vi "ServoTurn.vi"(4 "error in":errorcluster, 5 "Turn to":i16(ring)=-90 items=["-90°"=-90, "0°"=0, "+90°"=90], 6 "Servo Enum":T9, 7 "PWM channel\n cluster":T8) -> (0 "error out":errorcluster, 3 "PWM Ref Out":T1)   [LabVIEW 2017]
uses:
  <vilib>/myRIO/Instrument Drivers/Onboard IO/PWM/typedefs/PWM Reference.ctl
  <vilib>/myRIO/Common/Instrument Driver Framework/Utilities/typedefs/myRIO Generic Hardware Reference.ctl
  <vilib>/myRIO/Common/Instrument Driver Framework/Utilities/typedefs/Hardware Version Enum.ctl
  <vilib>/myRIO/Common/Instrument Driver Framework/Utilities/typedefs/myRIO v1.0 Reference.ctl
  <vilib>/myRIO/Common/Instrument Driver Framework/Utilities/typedefs/Generic FPGA Reference.ctl
  <vilib>/myRIO/Common/Instrument Driver Framework/myRIO v1.0/PWM/typedefs/PWM Channels Enum.ctl
  <vilib>/myRIO/Instrument Drivers/Onboard IO/PWM/typedefs/PWM Configuration.ctl
  ServoEnumControl.ctl
  <vilib>/Utility/error.llb/Error Cluster From Error Code.vi
  <vilib>/myRIO/Common/Instrument Driver Framework/myRIO v1.0/PWM/vis/myRIO v1.0 Write PWM.vi
  <vilib>/myRIO/Instrument Drivers/Onboard IO/PWM/PWM.lvlib
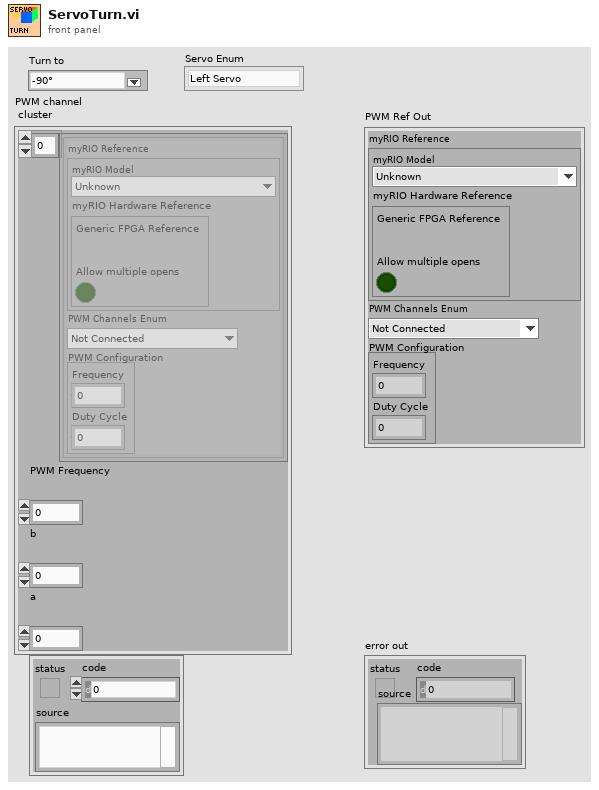
[diagram p1: front panel]
types:
  T1 = typedef "PWM.lvlib/PWM Reference.ctl" = cluster{"myRIO Reference":T2, "PWM Channels Enum":T6, "PWM Configuration":T7}
  T2 = typedef "myRIO Generic Hardware Reference.ctl" = cluster{"myRIO Model":T3, "myRIO Hardware Reference":T4}
  T3 = typedef "Hardware Version Enum.ctl" = enum16{"Unknown", "myRIO-1900", "myRIO-1950", "roboRIO", "NI ELVIS RIO CM"}
  T4 = typedef "myRIO v1.0 Reference.ctl" = cluster{"Generic FPGA Reference":T5, "Allow multiple opens":bool}
  T5 = typedef "Generic FPGA Reference.ctl" = refnum<k20>
  T6 = typedef "PWM Channels Enum.ctl" = enum16{"Not Connected", "C/PWM0", "C/PWM1", "A/PWM0", "A/PWM1", "A/PWM2", "B/PWM0", "B/PWM1", "B/PWM2", "PWM/PWM0", "PWM/PWM1", "PWM/PWM2", "PWM/PWM3", "PWM/PWM4", "PWM/PWM5", "PWM/PWM6", "PWM/PWM7", "PWM/PWM8", "PWM/PWM9"}
  T7 = typedef "PWM.lvlib/PWM Configuration.ctl" = cluster{"Frequency":dbl, "Duty Cycle":dbl}
  T8 = cluster{T1[], "PWM Frequency":dbl, "b":dbl, "a":dbl}
  T9 = typedef "ServoEnumControl.ctl" = enum16{"Left Servo", "Front Servo", "Right Servo"}
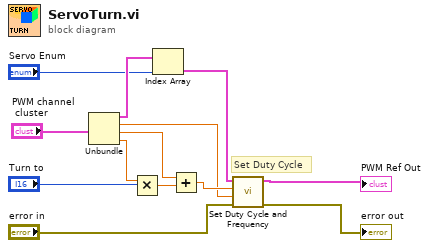
[diagram p0: block diagram]
diagram:
  # "Set Duty Cycle"
  n1 = Unbundle("PWM channel\n cluster") -> (w3:T1[], "PWM Frequency"=w4:dbl, "b"=w5:dbl, "a"=w6:dbl)
  n2 = Multiply(x=w6, y="Turn to") -> (x*y=w10:dbl)
  n3 = Index Array(array=w3, index="Servo Enum") -> (element=w1:T1)
  n4 = Add(x=w5, y=w10) -> (x+y=w9:dbl)
  n5 = call <vilib>:"Set Duty Cycle and Frequency.vi"("error in (no error)"="error in", "Frequency [Hz]"=w4, "Duty Cycle"=w9, "PWM Ref In"=w1) -> ("error out"=→"error out":errorcluster, "PWM Ref Out"=→"PWM Ref Out":T1)  [unwired: 5 in]
